vi "OpenShortDeembed.vi"(0 "Extrinsic DUT S-parameter Trace Array":T1(array[cluster])=[{"Freq (Hz)"=5000000.0, "S-parameter Array"=[[0.0+0.0i, 0.999+0.0i], [0.999+0.0i, 0.0+0.0i]]}] {"Freq (Hz)" format="%.2e"; "S-parameter Array" format="%.3f"}, 1 "Open S-parameter Trace Array":T1(array[cluster])=[{"Freq (Hz)"=5000000.0, "S-parameter Array"=[[0.999+0.0i, 0.0+0.0i], [0.0+0.0i, 0.999+0.0i]]}] {"Freq (Hz)" format="%.2e"; "S-parameter Array" format="%.3f"}, 2 "Short S-parameter Trace Array":T1(array[cluster])=[{"Freq (Hz)"=5000000.0, "S-parameter Array"=[[-0.999+0.0i, 0.0+0.0i], [0.0+0.0i, -0.999+0.0i]]}] {"Freq (Hz)" format="%.2e"; "S-parameter Array" format="%.3f"}, 3 "error in (no error)":errorcluster, 4 "Reference Impedance":dbl=50.0) -> (5 "Intrinsic DUT S-parameter Trace Array":T1(array[cluster])=[{"Freq (Hz)"=5000000.0, "S-parameter Array"=[[0.0+0.0i, 1.0+0.0i], [1.0+0.0i, 0.0+0.0i]]}] {"Freq (Hz)" format="%.2e"; "S-parameter Array" format="%.3f"}, 6 "error out":errorcluster)   [LabVIEW 2017]
uses:
  <vilib>/Analysis/baseanly.llb/Complex Inverse Matrix.vi
  <vilib>/Analysis/Matrix/Numeric/Subtract/Subtract - CM,CM.vi
  <vilib>/Analysis/NI_AALBase.lvlib
  <vilib>/Analysis/Matrix/NI_Matrix.lvlib
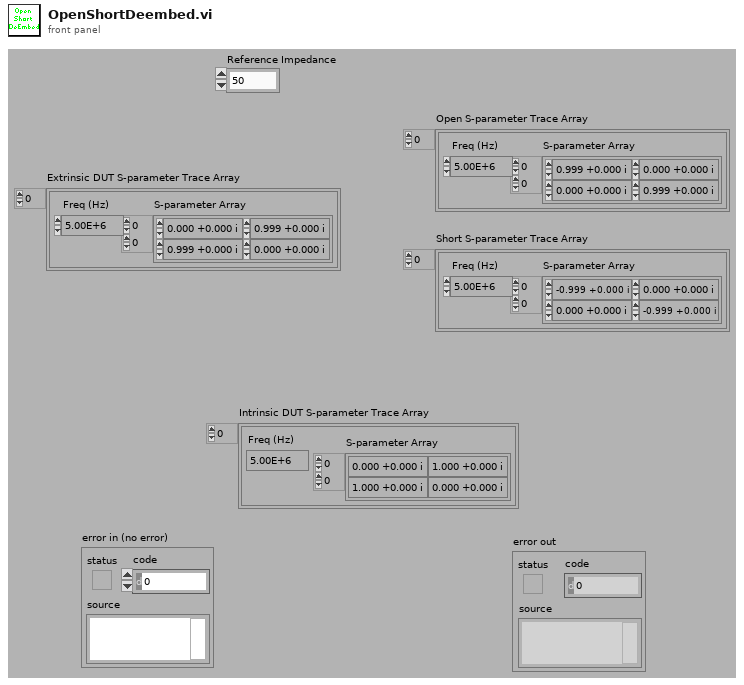
[diagram p1: front panel]
types:
  T1 = cluster{"Freq (Hz)":dbl, "S-parameter Array":csg[][]}[]
  T2 = cluster{"Freq (Hz)":dbl, "Y-parameter Array":csg[][]}[]
  T3 = typedef "NI_Matrix.lvlib/ComplexMatrix.ctl" = cdb[][]
  T4 = cluster{"Freq (Hz)":dbl, "Y-parameter Array":csg[][]}
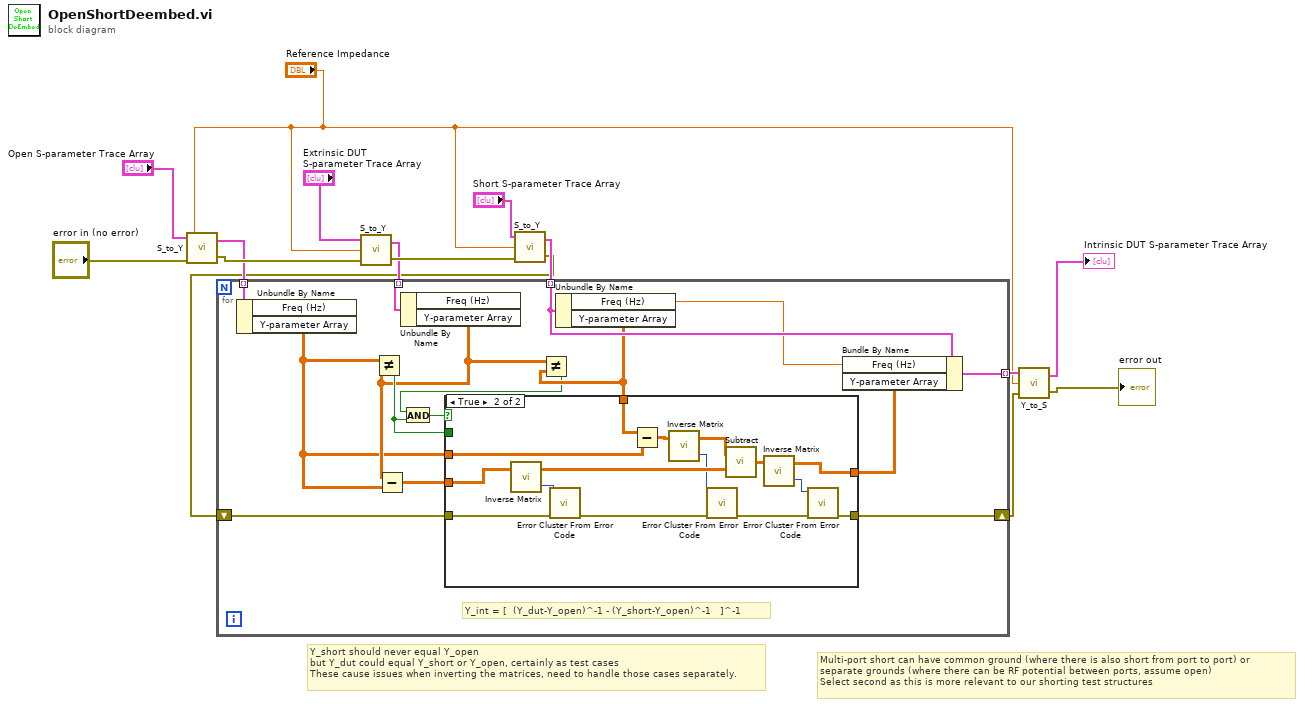
[diagram p0: block diagram]
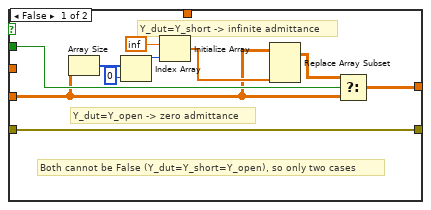
[diagram p2: hidden frame]
diagram:
  # "Multi-port short can have common ground (where there is also short from port to port) or\nseparate grounds (where there can be RF potential between ports, assume open)\nSelect second as this is more relevant to our shorting test structures"
  # "Y_short should never equal Y_open\nbut Y_dut could equal Y_short or Y_open, certainly as test cases\nThese cause issues when inverting the matrices, need to handle those cases separately."
  n1 = call "S_to_Y.vi"("error in (no error)"="error in (no error)", "Reference Impedance"="Reference Impedance", "Input S-parameter Trace Array"="Open S-parameter Trace Array") -> ("error out"=w11:errorcluster, "Output Y-parameter Trace Array"=w9:T2)
  n2 = call "S_to_Y.vi"("error in (no error)"=w11, "Reference Impedance"="Reference Impedance", "Input S-parameter Trace Array"="Extrinsic DUT S-parameter Trace Array") -> ("error out"=w10:errorcluster, "Output Y-parameter Trace Array"=w8:T2)
  n3 = call "S_to_Y.vi"("error in (no error)"=w10, "Reference Impedance"="Reference Impedance", "Input S-parameter Trace Array"="Short S-parameter Trace Array") -> ("error out"=w4:errorcluster, "Output Y-parameter Trace Array"=w7:T2)
  n4 = for {
    tunnel: w9 -> [w30] mode=indexing
    tunnel: w8 -> [w29] mode=indexing
    tunnel: w7 -> [w28] mode=indexing
    tunnel: [w26] -> w6 mode=indexing
    shift-right: [w25] -> w5
    shift-left: w4 -> [w24]
    # "Y_int = [  (Y_dut-Y_open)^-1 - (Y_short-Y_open)^-1   ]^-1"
    n5 = Unbundle By Name(w30) -> ("Y-parameter Array"=w17:csg[][])  [unwired: 1 out]
    n6 = Unbundle By Name(w29) -> ("Y-parameter Array"=w18:csg[][])  [unwired: 1 out]
    n7 = Not Equal?(x=w17, y=w18) -> (x != y?=w19:bool)
    n8 = Subtract(x=w18, y=w17) -> (x-y=w16:csg[][])
    n9 = Unbundle By Name(w28) -> ("Freq (Hz)"=w23:dbl, "Y-parameter Array"=w22:csg[][])
    n10 = Not Equal?(x=w18, y=w22) -> (x != y?=w20:bool)
    n11 = And(x=w20, y=w19) -> (x .and. y?=w21:bool)
    n12 = case shown="True" w21 {
      tunnel: w17 -> [_ w55]
      tunnel: w22 -> [_ w54]
      tunnel: [w39 w44] -> w27
      tunnel: [w38 w43] -> w25
      tunnel: w24 -> [w38 w42]
      tunnel: w19 -> [w40 _]
      tunnel: w16 -> [w31 w41]
      frame False {
        # "Y_dut=Y_short -> infinite admittance"
        # "Y_dut=Y_open -> zero admittance"
        # "Both cannot be False (Y_dut=Y_short=Y_open), so only two cases"
        n13 = Array Size(array=w31) -> (size(s)=w36:i32[])
        n14 = Index Array(array=w36, index=0) -> (element=w35:i32)
        n15 = Initialize Array(inf, w35) -> (w33:dbl[])
        n16 = Replace Array Subset(array=w31, new element=w33) -> (w32:T3)  [unwired: 2 in]
        n17 = Select(t=w32, s=w40, f=w31) -> (s? t:f=w39:T3)
      }
      frame True {
        n18 = call-poly <vilib>:"Inverse Matrix.vi"("Input Matrix"=w41) -> ("error"=w45:i32, "Inverse Matrix"=w51:T3)  [unwired: 1 in]
        n19 = call <vilib>:"Error Cluster From Error Code.vi"("error in (no error)"=w42, "error code (0)"=w45) -> ("error out"=w49:errorcluster)  [unwired: 1 in, 6 out]
        n20 = Subtract(x=w54, y=w55) -> (x-y=w53:csg[][])
        n21 = call-poly <vilib>:"Inverse Matrix.vi"("Input Matrix"=w53) -> ("error"=w46:i32, "Inverse Matrix"=w52:T3)  [unwired: 1 in]
        n22 = call <vilib>:"Error Cluster From Error Code.vi"("error in (no error)"=w49, "error code (0)"=w46) -> ("error out"=w48:errorcluster)  [unwired: 1 in, 6 out]
        n23 = call-poly <vilib>:"Subtract.vi"("Complex Matrix B"=w51, "Complex Matrix A"=w52) -> ("A - B"=w50:T3)
        n24 = call-poly <vilib>:"Inverse Matrix.vi"("Input Matrix"=w50) -> ("error"=w47:i32, "Inverse Matrix"=w44:T3)  [unwired: 1 in]
        n25 = call <vilib>:"Error Cluster From Error Code.vi"("error in (no error)"=w48, "error code (0)"=w47) -> ("error out"=w43:errorcluster)  [unwired: 1 in, 6 out]
      }
    }
    n26 = Bundle By Name(cluster=w28, "Freq (Hz)"=w23, "Y-parameter Array"=w27) -> (w26:T4)
  }
  n27 = call "Y_to_S.vi"("error in (no error)"=w5, "Reference Impedance"="Reference Impedance", "Input Y-parameter Trace Array"=w6) -> ("error out"=→"error out":errorcluster, "Output S-parameter Trace Array"=→"Intrinsic DUT S-parameter Trace Array":T1)
